vi "Low_Rank_Matrix.vi"(8 "error in (no error)":errorcluster caption="entrée d'erreur (pas d'erreur)", 11 "make_low_rank_matrix":T2={"n_samples"=100, "n_features"=100, "effective_rank"=10, "tail_strength"=0.5, "random_state"=-1} {"random_state" min=-1; "tail_strength" min=0.0 max=1.0; "n_features" min=1; "n_samples" min=1}) -> (0 "error out":errorcluster, 3 "Data":T1)   [LabVIEW 2020]
doc: "Generate a mostly low rank matrix with bell-shaped singular values\n\nMost of the variance can be explained by a bell-shaped curve of width effective_rank: the low rank part of the singular values profile is :\n (1 - tail_strength) * exp(-1.0 * (i / effective_rank) ** 2)\n\nThe remaining singular values’ tail is fat, decreasing as :\n\n tail_strength * exp(-0.1 * i / effective_rank)\n\nThe low rank part of the profile can be considered the structured signal part of the data while the tail can be considered the noisy part of the data that cannot be summarized by a low number of linear components (singular vectors).\n\nThis kind of singular profiles is often seen in practice, for instance :\n \n - gray level pictures of faces\n\n - TF-IDF vectors of text documents crawled from the web\n\n\n\nParameters :\n\n- n_samples : int, optional (default=100)\nThe number of samples.\n\n- n_features : int, optional (default=100)\nThe number of features.\n\n- effective_rank : int, optional (default=10)\nThe approximate number of singular vectors required to explain most of the data by linear combinations.\n\n- tail_strength : float between 0.0 and 1.0, optional (default=0.5)\nThe relative importance of the fat noisy tail of the singular values profile.\n\n- random_state : int, RandomState instance, default=None=-1\nDetermines random number generation for dataset creation. Pass an int for reproducible output across multiple function calls. See Glossary.\n\nReturns : \n\n-X : array of shape [n_samples, n_features]\nThe matrix."
uses:
  Low_Rank_Matrix.lvclass
panel:
  out "Low_Rank_Matrix.lvclass":refnum<class "Low_Rank_Matrix.lvclass">
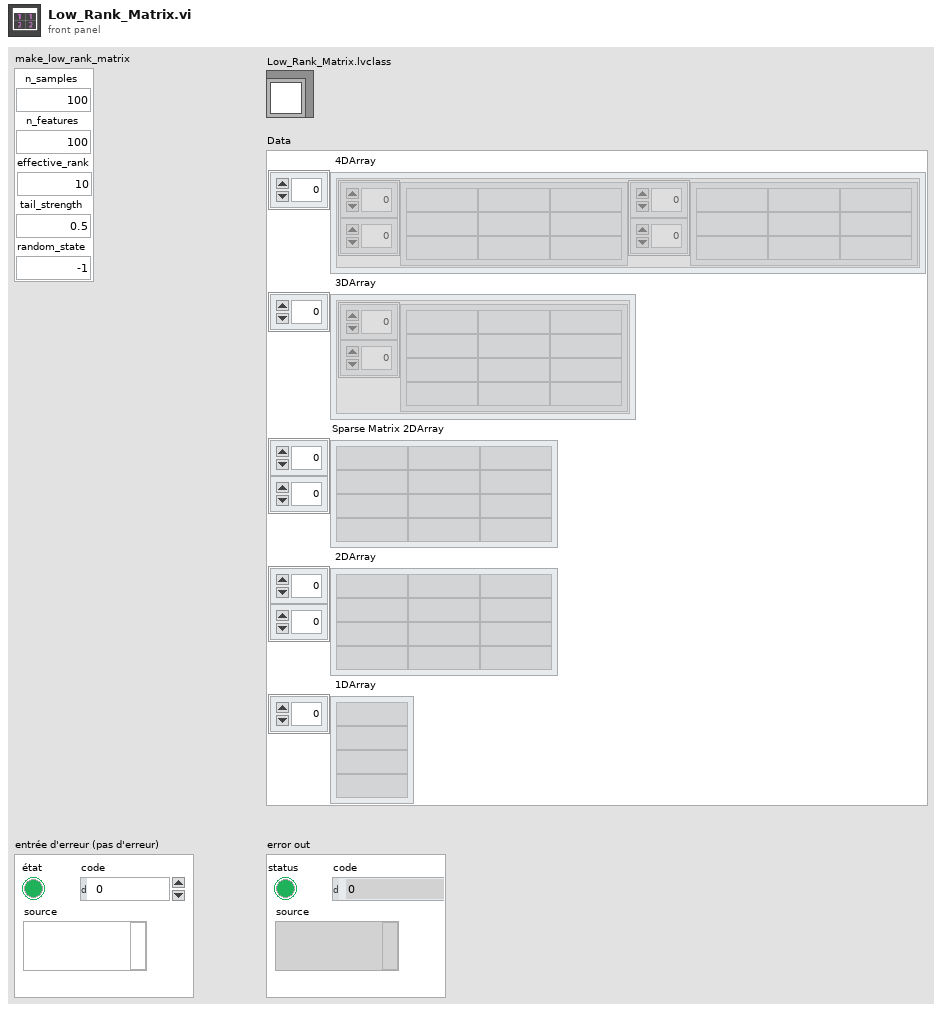
[diagram p1: front panel]
types:
  T1 = cluster{" 4DArray":cluster{"1":string[][], "2":string[][]}[], " 3DArray":cluster{"Tableau":string[][]}[], "Sparse Matrix 2DArray":string[][], " 2DArray":string[][], " 1DArray":string[]}
  T2 = cluster{"n_samples":u32, "n_features":u32, "effective_rank":i32, "tail_strength":dbl, "random_state":i32}
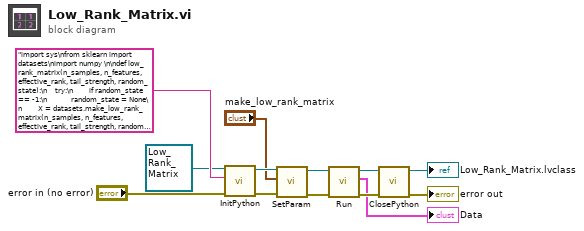
[diagram p0: block diagram]
diagram:
  n1 = call-dynamic "InitPython.vi"("error in (no error)"="error in (no error)", "Python Instruction"="import sys\nfrom sklearn import datasets\nimport numpy \n\ndef low_rank_matrix(n_samples, n_features, effective_rank, tail_strength, random_state):\n    try:\n        if random_state == -1:\n            random_state = None\n        X = datasets.make_low_rank_matrix(n_samples, n_features, effective_rank, tail_strength, random_state)\n        data = X.tolist()\n        return str(data)\n    except:\n        erreur = sys.exc_info()\n        typerr = u\"%s\" % (erreur[0])\n        typerr = typerr[typerr.find(\"'\")+1:typerr.rfind(\"'\")]\n        msgerr = u\"%s\" % (erreur[1])\n        message = str('/!\\\\ {0} : {1}'. format(typerr,msgerr))\n        return message", "Scikit-learn en entrée"=refnum<class "Low_Rank_Matrix.lvclass"> refnum ("Low_Rank_Matrix.lvclass")) -> ("error out"=w9:errorcluster, "Scikit-learn en sortie"=w10:refnum<class "Low_Rank_Matrix.lvclass">)  [unwired: 7 in]
  n2 = call-dynamic "SetParam.vi"("error in (no error)"=w9, "make_low_rank_matrix"="make_low_rank_matrix", "Low_Rank_Matrix.lvclass"=w10) -> ("error out"=w6:errorcluster, "Low_Rank_Matrix.lvclass"=w7:refnum<class "Low_Rank_Matrix.lvclass">)  [unwired: 7 in]
  n3 = call-dynamic "Run.vi"("error in (no error)"=w6, "Low_Rank_Matrix.lvclass"=w7) -> ("error out"=w4:errorcluster, "Data"=→"Data":T1, "Low_Rank_Matrix.lvclass"=w5:refnum<class "Low_Rank_Matrix.lvclass">)  [unwired: 7 in]
  n4 = call-dynamic "ClosePython.vi"("error in (no error)"=w4, "Scikit-learn en entrée"=w5) -> ("error out"=→"error out":errorcluster, "Scikit-learn en sortie"=→"Low_Rank_Matrix.lvclass":refnum<class "Low_Rank_Matrix.lvclass">)  [unwired: 8 in]
